vi "Name_Piezo_Disc.vi"() -> (2 "PZT path out":path)   [LabVIEW 2012]
uses:
  <vilib>/Utility/sysdir.llb/System Directory Type.ctl
panel:
  in  "piezo name":string
  in  "OK Button":bool
  # "Please give this piezo disc a name:"
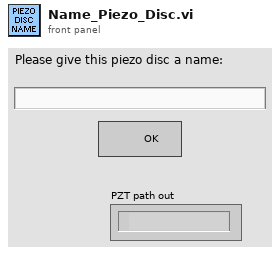
[diagram p1: front panel]
types:
  T1 = typedef "System Directory Type.ctl" = i32
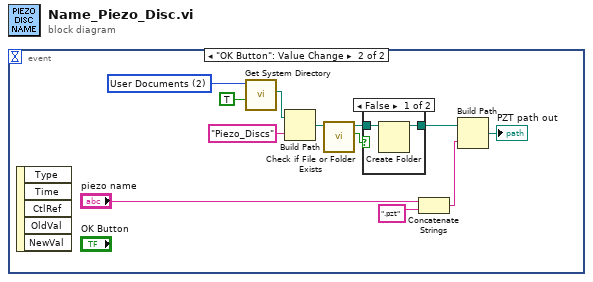
[diagram p0: block diagram]
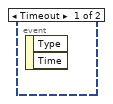
[diagram p2: hidden frame]
diagram:
  n1 = event shown="[1] \"OK Button\": Value Change" {
    selector: _ -> [_ _]
    dyn-events: _ -> [_ _]
    timeout: _ -> [_ _]
    event Timeout {
      n2 = event-data() -> ()  [unwired: 1 in, 2 out]
    }
    event "OK Button": Value Change {
      w11 = T1 2 items=["User Home"=0, "User Desktop"=1, "User Documents"=2, "User Application Data"=3, "User Preferences"=4, "User Temporary"=5, "Public Documents"=6, "Public Application Data"=7, "Public Preferences"=8, "Public Cache"=13, "System Core Libraries"=9, "System Installed Libraries"=10, "Application Files"=11, "Boot Volume Root"=12] ("system directory type")
      n3 = event-data() -> ()  [unwired: 1 in, 5 out]
      n4 = call <vilib>:"Get System Directory.vi"("create directory if not found? (F)"=TRUE, "system directory type"=w11) -> ("system directory"=w10:path)  [unwired: 9 in]
      n5 = Build Path(base path=w10, name or relative path="Piezo_Discs") -> (appended path=w6:path)
      n6 = call <vilib>:"Check if File or Folder Exists.vi"("path"=w6) -> ("file or folder exists?"=w5:bool, "dup path"=w3:path)  [unwired: 8 in, 1 out]
      n7 = case shown="False" w5 {
        tunnel: w3 -> [w14 w15]
        tunnel: [w13 w15] -> w2
        frame False {
          n8 = Create Folder(path (use dialog)=w14) -> (created path=w13:path)  [unwired: 2 in, 2 out]
        }
        frame True {
        }
      }
      n9 = Concatenate Strings("piezo name", ".pzt" ("string")) -> (w4:string)
      n10 = Build Path(base path=w2, name or relative path=w4) -> (appended path=→"PZT path out":path)
    }
  }
